vi "WhichTowerVisible.vi"(3 "No. of Goals":i32, 4 "X Position":dbl, 5 "Goal Measurements":dbl[][](array[numeric])) -> (0 "Goal C":cluster{"X":dbl, "Y":dbl, "Dist":dbl}, 1 "Goal B":cluster{"X":dbl, "Y":dbl, "Dist":dbl}, 2 "Goal A":cluster{"X":dbl, "Y":dbl, "Dist":dbl})   [LabVIEW 2015]
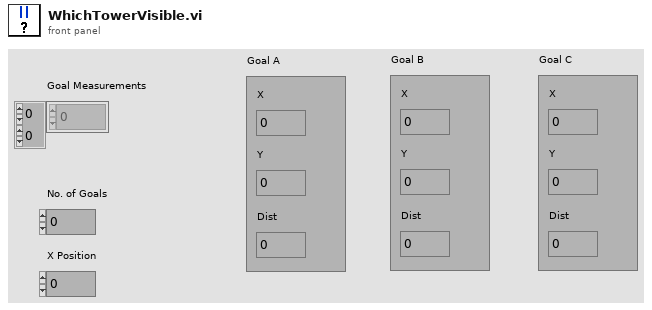
[diagram p1: front panel]
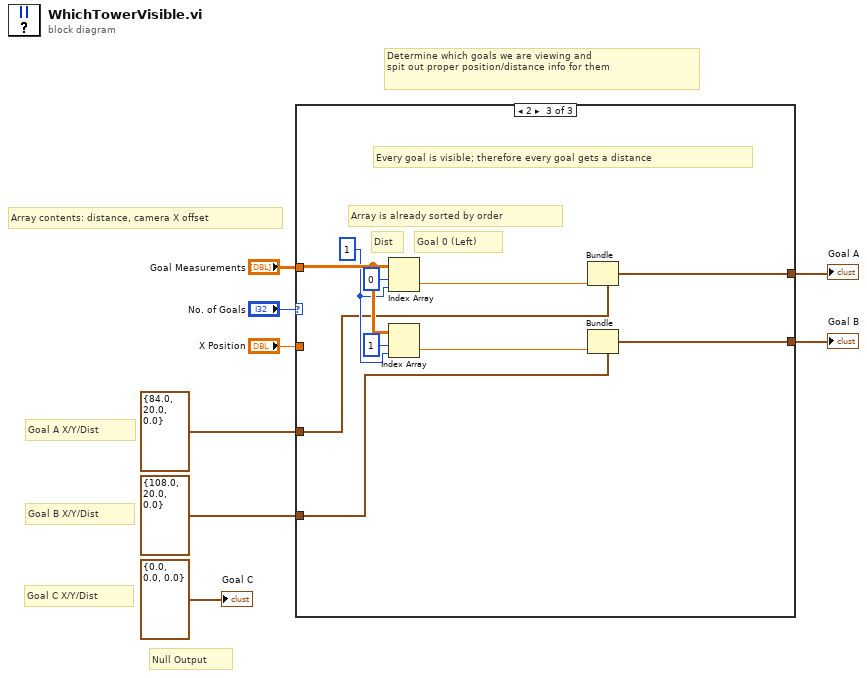
[diagram p0: block diagram]
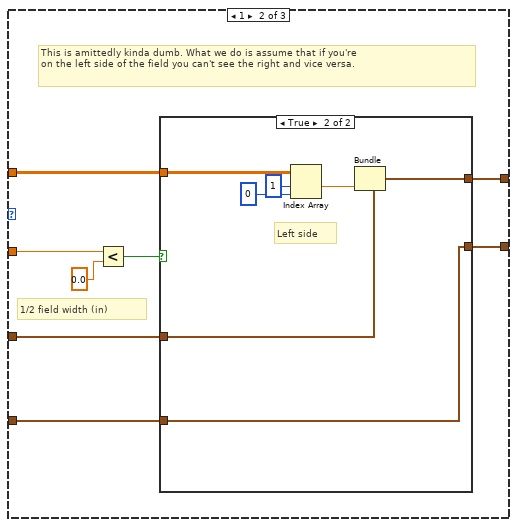
[diagram p3: hidden frame]
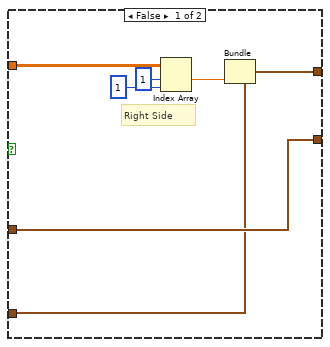
[diagram p4: hidden frame]
diagram:
  # "Array contents: distance, camera X offset"
  # "Null Output"
  # "Determine which goals we are viewing and\nspit out proper position/distance info for them"
  # "Goal C X/Y/Dist"
  # "Goal B X/Y/Dist"
  # "Goal A X/Y/Dist"
  n1 = case shown="2" "No. of Goals" {
    tunnel: [w10 w12 w40] -> w7
    tunnel: [w9 w13 w39] -> w6
    tunnel: "Goal Measurements" -> [_ w14 w42]
    tunnel: cluster{dbl, dbl, dbl} {84.0, 20.0, 0.0} -> [w10 w16 w35]
    tunnel: cluster{dbl, dbl, dbl} {108.0, 20.0, 0.0} -> [w9 w15 w34]
    tunnel: "X Position" -> [_ w11 _]
    frame 0, Default {
      # "There are no goals"
    }
    frame 1 {
      # "This is amittedly kinda dumb. What we do is assume that if you're\non the left side of the field you can't see the right and vice versa."
      # "1/2 field width (in)"
      n2 = Less?(x=w11, y=0.0) -> (x < y?=w17:bool)
      n3 = case shown="True" w17 {
        tunnel: w16 -> [w20 w29]
        tunnel: w15 -> [w19 w26]
        tunnel: w14 -> [w22 w32]
        tunnel: [w20 w26] -> w13
        tunnel: [w21 w27] -> w12
        frame False {
          # "Right Side"
          n4 = Index Array(array=w22, index (row)=1, index (col)=1 ("index (row)")) -> (element=w23:dbl)
          n5 = Bundle(cluster=w19, w23) -> (w21:cluster{dbl, dbl, dbl})  [unwired: 2 in]
        }
        frame True {
          # "Left side"
          n6 = Index Array(array=w32, index (row)=1, index (col)=0 ("index (row)")) -> (element=w28:dbl)
          n7 = Bundle(cluster=w29, w28) -> (w27:cluster{dbl, dbl, dbl})  [unwired: 2 in]
        }
      }
    }
    frame 2 {
      w36 = 1 ("index (col)")
      # "Every goal is visible; therefore every goal gets a distance"
      # "Goal 0 (Left)"
      # "Dist"
      # "Array is already sorted by order"
      n8 = Index Array(array=w42, index (row)=0, index (col)=w36) -> (element=w33:dbl)
      n9 = Index Array(array=w42, index (row)=1, index (col)=w36) -> (element=w38:dbl)
      n10 = Bundle(cluster=w35, w33) -> (w40:cluster{dbl, dbl, dbl})  [unwired: 2 in]
      n11 = Bundle(cluster=w34, w38) -> (w39:cluster{dbl, dbl, dbl})  [unwired: 2 in]
    }
  }
  "Goal A" <- w7
  "Goal B" <- w6
  "Goal C" <- cluster{dbl, dbl, dbl} {0.0, 0.0, 0.0}
